vi "TH_DateTime.vi"() -> (3 "Tid och Datum":string)   [LabVIEW 2020]
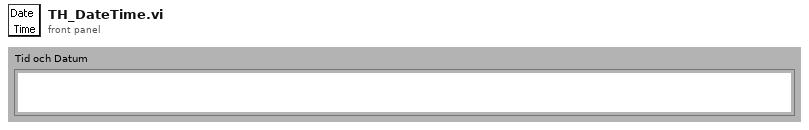
[diagram p1: front panel]
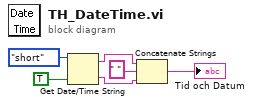
[diagram p0: block diagram]
diagram:
  n1 = Get Date/Time String(date format (0)=enum16{"short", "long", "abbreviated"}."short", want seconds? (F)=TRUE) -> (date string=w2:string, time string=w6:string)  [unwired: 1 in]
  n2 = Concatenate Strings(w2, " ", w6) -> (→"Tid och Datum":string)
